vi "Read Operatator Joystick.vi"(11 "Operator Joystick":T1) -> ()   [LabVIEW 2019]
uses:
  <vilib>/Rock Robotics/WPI/Joystick/WPI_JoystickDevRef.ctl
  <vilib>/Rock Robotics/WPI/Joystick/WPI_JoystickDeviceEnum.ctl
  Framework/Robot Global Data.vi
panel:
  # "READ OPERATOR JOYSTICK"
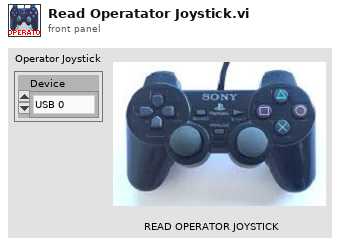
[diagram p1: front panel]
types:
  T1 = typedef "WPI_JoystickDevRef.ctl" = cluster{"Device":T2}
  T2 = typedef "WPI_JoystickDeviceEnum.ctl" = enum16{"USB 0", "USB 1", "USB 2", "USB 3", "USB 4", "USB 5"}
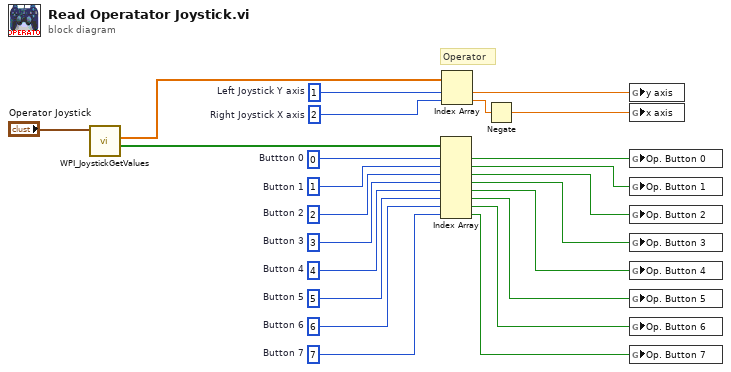
[diagram p0: block diagram]
diagram:
  w4 = 7  # Button 7
  w16 = 6  # Button 6
  w15 = 5  # Button 5
  w17 = 4  # Button 4
  w18 = 3  # Button 3
  w19 = 2  # Button 2
  w20 = 1  # Button 1
  w21 = 0  # Buttton 0
  w23 = 2  # Right Joystick X axis
  w24 = 1  # Left Joystick Y axis
  # "Operator"
  n1 = call <vilib>:"WPI_JoystickGetValues.vi"("JoystickDevRef"="Operator Joystick") -> ("Buttons"=w13:bool[], "Axes"=w12:dbl[])  [unwired: 6 in, 3 out]
  n2 = Index Array(array=w13, index #1=w21, index #2=w20, index #3=w19, index #4=w18, index #5=w17, index #6=w15, index #7=w16, index #8=w4) -> (element #1=w14:bool, element #2=w11:bool, element #3=w10:bool, element #4=w6:bool, element #5=w9:bool, element #6=w8:bool, element #7=w7:bool, element #8=w5:bool)
  n3 = Index Array(array=w12, index #1=w24, index #2=w23) -> (element #1=w3:dbl, element #2=w22:dbl)
  n4 = Negate(x=w22) -> (-x=w2:dbl)
  n5 = global write "Robot Global Data.vi" "y axis"(w3) -> ()
  n6 = global write "Robot Global Data.vi" "x axis"(w2) -> ()
  n7 = global write "Robot Global Data.vi" "Op. Button 0"(w14) -> ()
  n8 = global write "Robot Global Data.vi" "Op. Button 1"(w11) -> ()
  n9 = global write "Robot Global Data.vi" "Op. Button 2"(w10) -> ()
  n10 = global write "Robot Global Data.vi" "Op. Button 3"(w6) -> ()
  n11 = global write "Robot Global Data.vi" "Op. Button 4"(w9) -> ()
  n12 = global write "Robot Global Data.vi" "Op. Button 5"(w8) -> ()
  n13 = global write "Robot Global Data.vi" "Op. Button 6"(w7) -> ()
  n14 = global write "Robot Global Data.vi" "Op. Button 7"(w5) -> ()
